vi "Filter Control Drag Source Update Event.vi"(8 "error in (no error)":errorcluster, 10 "ControlDragSourceUpdateMsg":refnum<class "ControlDragSourceUpdateMsg.lvclass">, 11 "IEventFilter in":refnum<class "IEventFilter.lvclass">) -> (0 "error out":errorcluster, 1 "Discard?":bool, 2 "Filtered Event Data":cluster{"Cursor":refnum<k1>}, 3 "IEventFilter out":refnum<class "IEventFilter.lvclass">, 5 "Data Filtered?":bool)   [LabVIEW 2020, in "ActorEvents.lvlib" / "IEventFilter.lvclass"]
doc: "过滤控件数据源更新事件"
uses:
  IEventFilter.lvclass
  IEventAggregator Messages/ControlDragSourceUpdateMsg/ControlDragSourceUpdateMsg.lvclass
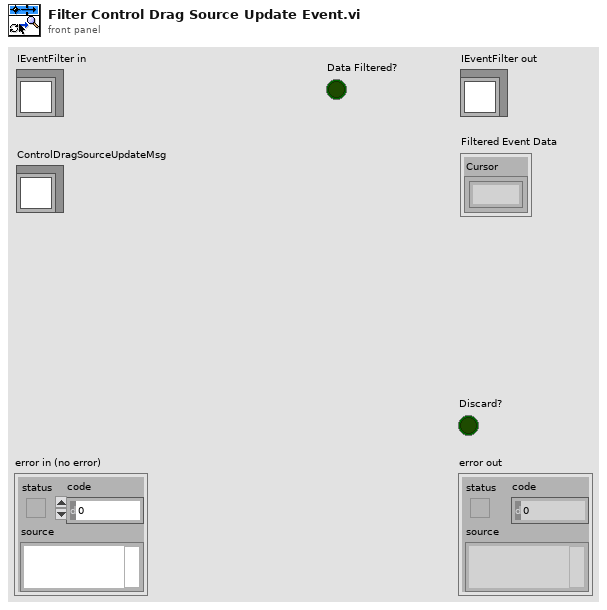
[diagram p1: front panel]
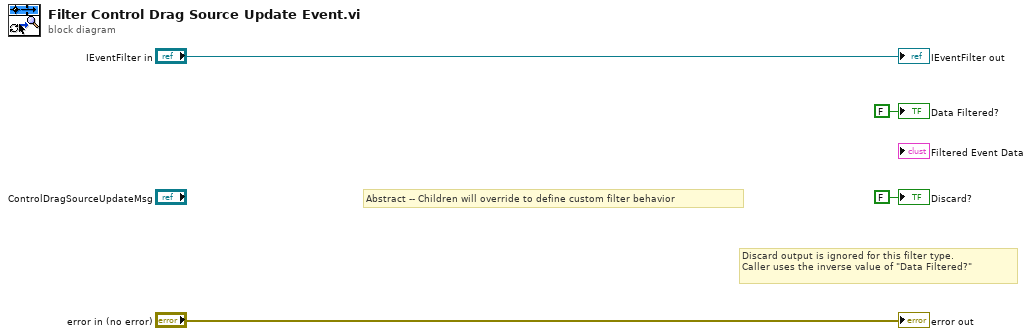
[diagram p0: block diagram]
diagram:
  # "Discard output is ignored for this filter type.\nCaller uses the inverse value of \"Data Filtered?\""
  # "Abstract -- Children will override to define custom filter behavior"
  "error out" <- "error in (no error)"
  "IEventFilter out" <- "IEventFilter in"
  "Discard?" <- FALSE ("Discard?")
  "Data Filtered?" <- FALSE ("Data Filtered?")
